vi "ALTS-2015 TTA TTB to Test Type.vi"(10 "TTB":bool, 11 "TTA":bool) -> (3 "Test Type":i32)   [LabVIEW 2013]
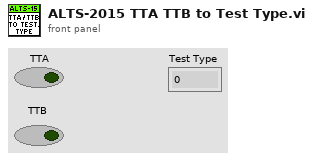
[diagram p1: front panel]
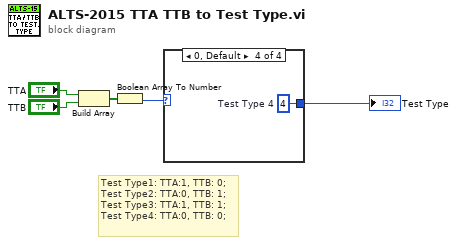
[diagram p0: block diagram]
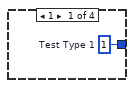
[diagram p2: hidden frame]
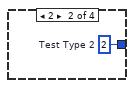
[diagram p3: hidden frame]
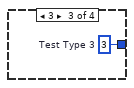
[diagram p4: hidden frame]
diagram:
  # "Test Type1: TTA:1, TTB: 0;\nTest Type2: TTA:0, TTB: 1;\nTest Type3: TTA:1, TTB: 1;\nTest Type4: TTA:0, TTB: 0;"
  n1 = Build Array("TTA", "TTB") -> (w1:bool[])
  n2 = Boolean Array To Number(Boolean array=w1) -> (number=w2:u32)
  n3 = case shown="0, Default" w2 {
    tunnel: [w6 w7 w8 w9] -> w5
    frame 1 {
      w6 = 1  # Test Type 1
    }
    frame 2 {
      w7 = 2  # Test Type 2
    }
    frame 3 {
      w8 = 3  # Test Type 3
    }
    frame 0, Default {
      w9 = 4  # Test Type 4
    }
  }
  "Test Type" <- w5
